vi "SAOMM-ROI_XY.vi"(0 "PRAMMS-COMM IN":refnum<visa-resource-name>="COM4", 1 "Active Refnum":refnum<vi>, 2 "PrAMS-ACK":refnum<vi>, 3 "MessageType":cluster{string[], u32[]}, 11 "Error IN":errorcluster, 12 "Offset X":u16, 13 "Offset Y":u16) -> (4 "PRAMMS-COMM OUT":refnum<visa-resource-name>="COM4", 8 "Error":bool, 15 "Error OUT":errorcluster)   [LabVIEW 2011]
uses:
  Polymorphics/Num2littleEndian(DBL).vi
  Polymorphics/Num2littleEndian(U16).vi
panel:
  in  "Reference Y":dbl
  in  "Reference X":dbl
  in  "Signature":u32=1886544237
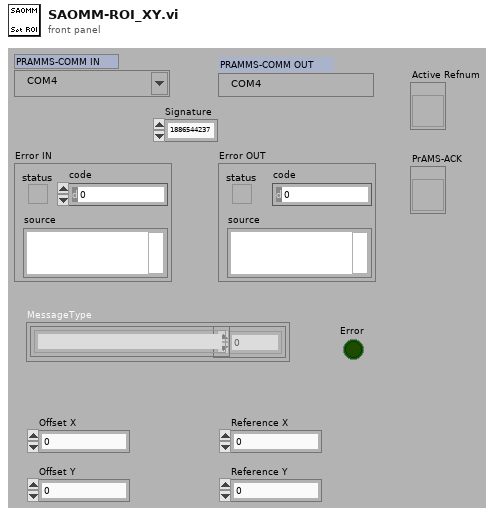
[diagram p1: front panel]
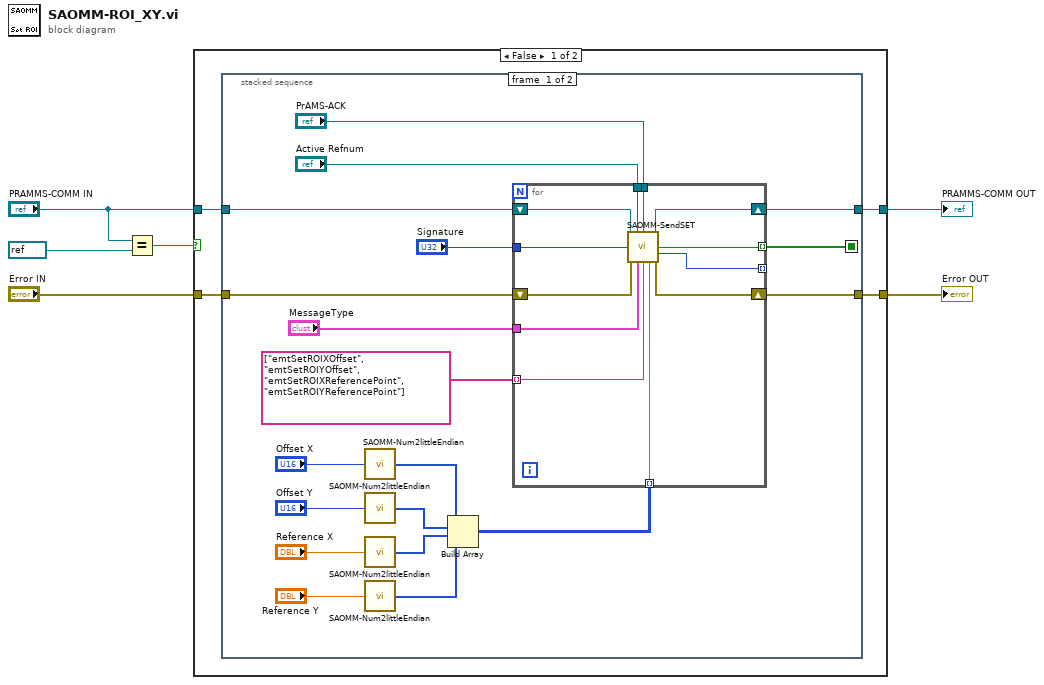
[diagram p0: block diagram]
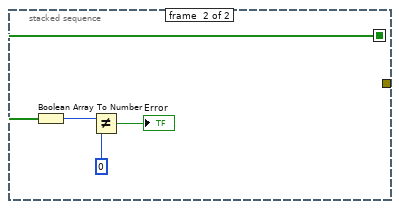
[diagram p2: hidden frame]
diagram:
  n1 = Equal?(x="PRAMMS-COMM IN", y=refnum<visa-resource-name> "-1") -> (x = y?=w5:bool)
  n2 = case shown="False" w5 {
    tunnel: "PRAMMS-COMM IN" -> [w10 w47]
    tunnel: "Error IN" -> [w9 w46]
    tunnel: [w8 w47] -> w2
    tunnel: [w7 w46] -> w1
    frame False {
      n3 = stacked-sequence {
        seq-local: [w22 _] -> [_ w45]
        tunnel: w10 -> [w28 _]
        tunnel: w9 -> [w27 _]
        tunnel: [w26 _] -> w8
        tunnel: [w25 _] -> w7
        frame #0 {
          n4 = call-poly "SAOMM-Num2littleEndian.vi"("Number"="Offset X") -> ("LiitleEndianedData"=w18:u8[])  [unwired: 14 in]
          n5 = call-poly "SAOMM-Num2littleEndian.vi"("Number"="Offset Y") -> ("LiitleEndianedData"=w16:u8[])  [unwired: 14 in]
          n6 = call-poly "SAOMM-Num2littleEndian.vi"("Number"="Reference X") -> ("LiitleEndianedData"=w12:u8[])  [unwired: 14 in]
          n7 = call-poly "SAOMM-Num2littleEndian.vi"("Number"="Reference Y") -> ("LiitleEndianedData"=w11:u8[])  [unwired: 14 in]
          n8 = Build Array(w18, w16, w12, w11) -> (w29:u8[][])
          n9 = for {
            tunnel: w29 -> [w34] mode=indexing
            shift-right: [w39] -> w26
            shift-left: w28 -> [w40]
            shift-right: [w38] -> w25
            shift-left: w27 -> [w41]
            tunnel: string[] ["emtSetROIXOffset", "emtSetROIYOffset", "emtSetROIXReferencePoint", "emtSetROIYReferencePoint"] -> [w35] mode=indexing
            tunnel: "PrAMS-ACK" -> [w36]
            tunnel: "Active Refnum" -> [w37]
            tunnel: [w33] -> w22 mode=indexing
            tunnel: "MessageType" -> [w32]
            tunnel: "Signature" -> [w31]
            tunnel: [w30] -> _ mode=indexing
            n10 = call "SAOMM-SendSET.vi"("PRAMMS-COMM IN"=w40, "Active Refnum"=w37, "PrAMS-ACK"=w36, "Signature"=w31, "Error IN"=w41, "MessageType"=w32, "Active SET"=w35, "Value (little endianed byte array)"=w34) -> ("PRAMMS-COMM OUT"=w39:refnum<visa-resource-name>, "Error"=w33:bool, "WaitACKTime"=w30:u32, "Error OUT"=w38:errorcluster)  [unwired: 4 in]
          }
        }
        frame #1 {
          n11 = Boolean Array To Number(Boolean array=w45) -> (number=w44:u32)
          n12 = Not Equal?(x=w44, y=u32 0) -> (x != y?=→"Error":bool)
        }
      }
    }
    frame True {
    }
  }
  "Error OUT" <- w1
  "PRAMMS-COMM OUT" <- w2
